vi "Get DT Cells in Opp. Target Range.vi"(0 "Parsed Board Info":T1, 1 "Danger Free DT Cells":i32[](array[numeric])) -> (12 "Empty?":bool, 14 "Intended Array":i32[](array[numeric]), 15 "DT Cells in Opp. Target Range":i32[](array[numeric]))   [LabVIEW 2014]
uses:
  Typedefs/Parsed Board.ctl
  Dragon Tamers.lvlib
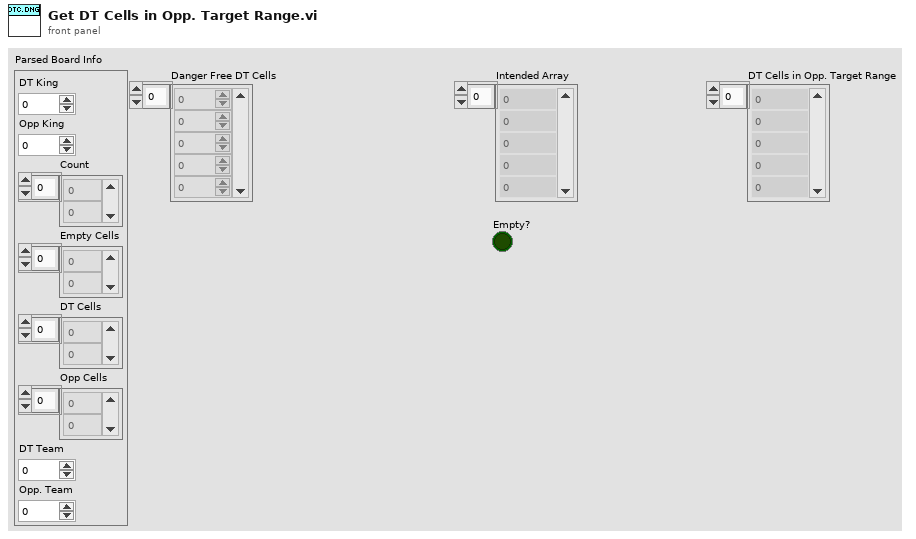
[diagram p1: front panel]
types:
  T1 = typedef "Dragon Tamers.lvlib/Parsed Board.ctl" = cluster{"DT King":i32, "Opp King":i32, "Count":i32[], "Empty Cells":i32[], "DT Cells":i32[], "Opp Cells":i32[], "DT Team":i32, "Opp. Team":i32}
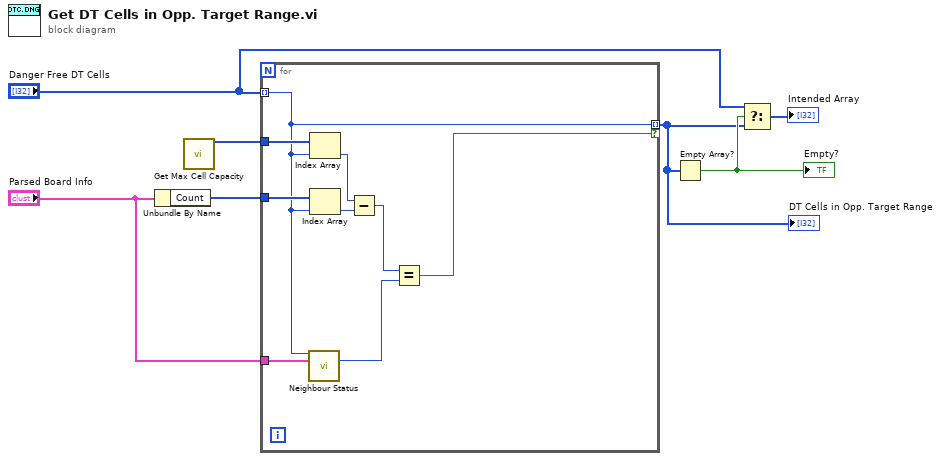
[diagram p0: block diagram]
diagram:
  n1 = Unbundle By Name("Parsed Board Info") -> ("Count"=w3:i32[])
  n2 = call "Get Max Cell Capacity.vi"() -> ("Max Capacity[]"=w2:i32[])  [unwired: 14 in, 1 out]
  n3 = for {
    tunnel: "Danger Free DT Cells" -> [w13] mode=indexing
    tunnel: [w13] -> w5 mode=indexing if=w8
    tunnel: "Parsed Board Info" -> [w16]
    tunnel: w3 -> [w15]
    tunnel: w2 -> [w14]
    n4 = call "Neighbour Status.vi"("Cell"=w13, "Parsed Board"=w16) -> ("Min Count to Max"=w9:i32)  [unwired: 10 in, 3 out]
    n5 = Index Array(array=w14, index=w13) -> (element=w12:i32)
    n6 = Index Array(array=w15, index=w13) -> (element=w11:i32)
    n7 = Subtract(x=w12, y=w11) -> (x-y=w10:i32)
    n8 = Equal?(x=w10, y=w9) -> (x = y?=w8:bool)
  }
  "DT Cells in Opp. Target Range" <- w5
  n9 = Empty Array?(array=w5) -> (empty?=w7:bool)
  "Empty?" <- w7
  n10 = Select(t="Danger Free DT Cells", s=w7, f=w5) -> (s? t:f=→"Intended Array":i32[])
